vi "Get Shared File Paths.vi"() -> (2 "Hardware File":path, 3 "Parameters File":path)   [LabVIEW 2020]
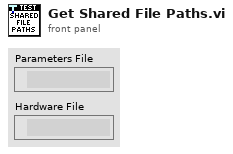
[diagram p1: front panel]
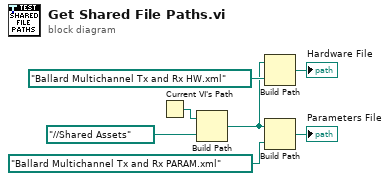
[diagram p0: block diagram]
diagram:
  n1 = Current VI's Path() -> (path=w1:path)
  n2 = Build Path(base path=w1, name or relative path=path "../../Shared Assets") -> (appended path=w4:path)
  n3 = Build Path(base path=w4, name or relative path=path "Ballard Multichannel Tx and Rx HW.xml") -> (appended path=→"Hardware File":path)
  n4 = Build Path(base path=w4, name or relative path=path "Ballard Multichannel Tx and Rx PARAM.xml") -> (appended path=→"Parameters File":path)
